vi "frw_extra_elements.vi"(9 "single field":string, 10 "fields":string[](array[string]), 11 "string":string) -> (0 "values":string[](array[string]), 1 "#ch":i32, 2 "fs":i32, 3 "data_format":string, 4 "single string":string)   [LabVIEW 2013]
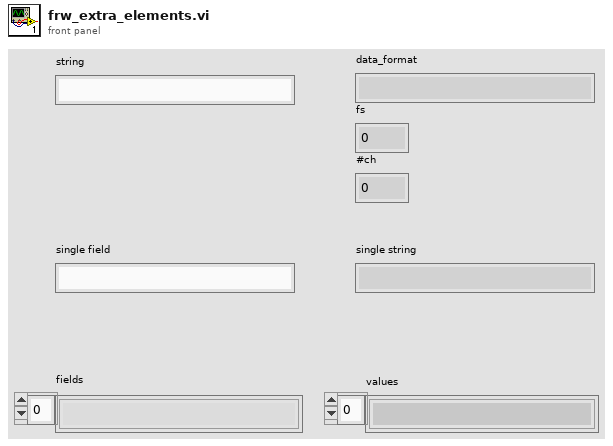
[diagram p1: front panel]
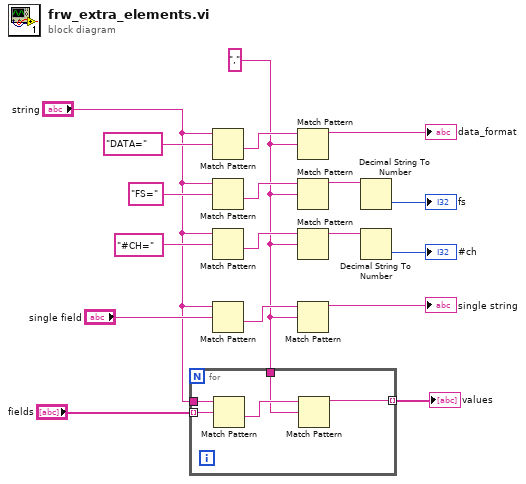
[diagram p0: block diagram]
diagram:
  w3 = ","
  n1 = for {
    tunnel: "string" -> [w22]
    tunnel: "fields" -> [w21] mode=indexing
    tunnel: w3 -> [w20]
    tunnel: [w19] -> w10 mode=indexing
    n2 = Match Pattern(string=w22, regular expression=w21) -> (after substring=w23:string)  [unwired: 1 in, 3 out]
    n3 = Match Pattern(string=w23, regular expression=w20) -> (before substring=w19:string)  [unwired: 1 in, 3 out]
  }
  "values" <- w10
  n4 = Match Pattern(string="string", regular expression="DATA=" ("delimiter (Tab)")) -> (after substring=w18:string)  [unwired: 1 in, 3 out]
  n5 = Match Pattern(string="string", regular expression="FS=" ("delimiter (Tab)")) -> (after substring=w16:string)  [unwired: 1 in, 3 out]
  n6 = Match Pattern(string="string", regular expression="#CH=" ("delimiter (Tab)")) -> (after substring=w15:string)  [unwired: 1 in, 3 out]
  n7 = Match Pattern(string="string", regular expression="single field") -> (after substring=w4:string)  [unwired: 1 in, 3 out]
  n8 = Match Pattern(string=w18, regular expression=w3) -> (before substring=→"data_format":string)  [unwired: 1 in, 3 out]
  n9 = Match Pattern(string=w16, regular expression=w3) -> (before substring=w9:string)  [unwired: 1 in, 3 out]
  n10 = Match Pattern(string=w15, regular expression=w3) -> (before substring=w7:string)  [unwired: 1 in, 3 out]
  n11 = Match Pattern(string=w4, regular expression=w3) -> (before substring=→"single string":string)  [unwired: 1 in, 3 out]
  n12 = Decimal String To Number(string=w9) -> (number=→"fs":i32)  [unwired: 2 in, 1 out]
  n13 = Decimal String To Number(string=w7) -> (number=→"#ch":i32)  [unwired: 2 in, 1 out]
